vi "Write Note.vi"(10 "Note":string, 11 "S Parameter in":refnum<class "S Parameter.lvclass">) -> (3 "S Parameter out":refnum<class "S Parameter.lvclass">)   [LabVIEW 2020, in "S Parameter.lvclass"]
uses:
  S Parameter.lvclass
  S Parameter.lvclass/S Parameter.ctl
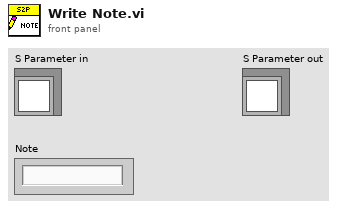
[diagram p1: front panel]
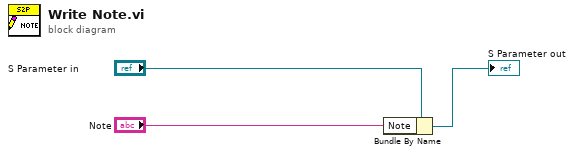
[diagram p0: block diagram]
diagram:
  n1 = Bundle By Name(cluster="S Parameter in", "Note"="Note") -> (→"S Parameter out":refnum<class "S Parameter.lvclass">)
